vi "GenerateCalibrationSequence.vi"(8 "Pressure Group":u8[](array[numeric])=[3, 3, 3, 3, 4, 4, 4, 4], 11 "Mix Cluster":T1={"Ratio"=[0.6, 0.6, 0.6, 0.6, 0.6, 0.6, 0.6, 0.6], "Mix 2"=[8, 8], "Mix 1"=[0, 0]} {"Mix 1" items=["A1"=0, "A2"=1, "A3"=2, "A4"=3, "A5"=12]; "Mix 2" items=["B5"=8, "B6"=9, "B7"=10, "B8"=11, "A5"=12]}) -> (3 "Calibration Refs":T2)   [LabVIEW 2016]
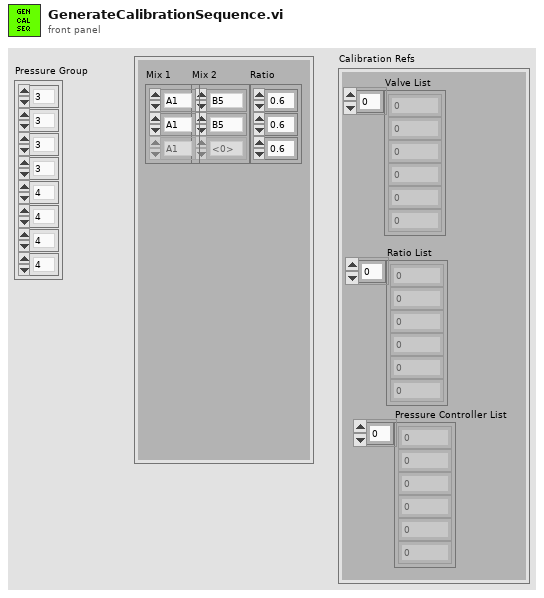
[diagram p1: front panel]
types:
  T1 = cluster{"Ratio":dbl[], "Mix 2":u16[], "Mix 1":u16[]}
  T2 = cluster{"Pressure Controller List":u8[], "Ratio List":dbl[], "Valve List":u16[]}
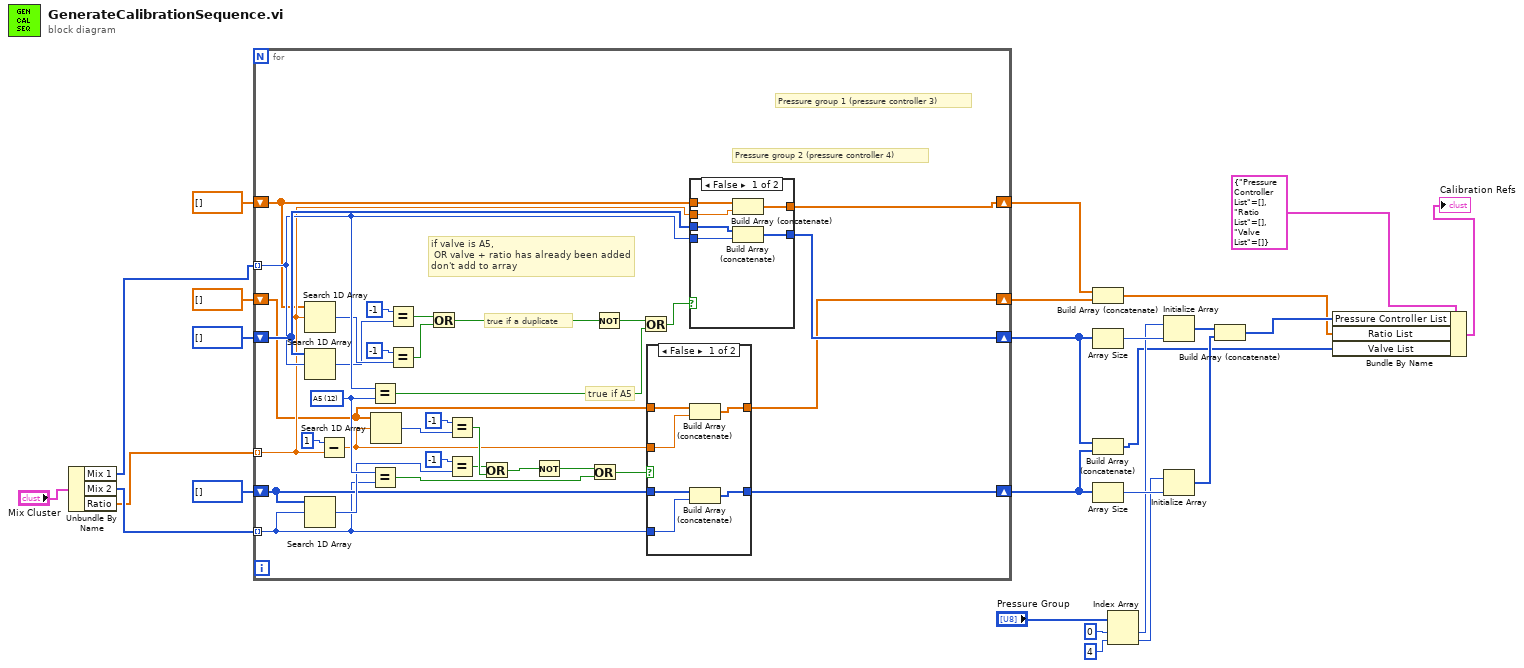
[diagram p0: block diagram]
diagram:
  n1 = Unbundle By Name("Mix Cluster") -> ("Mix 1"=w4:u16[], "Mix 2"=w3:u16[], "Ratio"=w2:dbl[])
  n2 = for {
    tunnel: w4 -> [w53] mode=indexing
    shift-right: [w60] -> w11
    shift-left: u16[] [] -> [w54]
    tunnel: w2 -> [w52] mode=indexing
    shift-right: [w56] -> w12
    shift-left: dbl[] [] -> [w51]
    tunnel: w3 -> [w33] mode=indexing
    shift-right: [w58] -> w13
    shift-left: dbl[] [] -> [w32]
    shift-right: [w57] -> w10
    shift-left: u16[] [] -> [w34]
    w55 = u16 12 items=["A1"=0, "A2"=1, "A3"=2, "A4"=3, "A5"=12] ("Ring")
    # "true if A5"
    # "true if a duplicate"
    # "if valve is A5,\n OR valve + ratio has already been added\ndon't add to array"
    # "Pressure group 2 (pressure controller 4)"
    # "Pressure group 1 (pressure controller 3)"
    n3 = Search 1D Array(1D array=w51, element=w52) -> (index of element=w50:i32)  [unwired: 1 in]
    n4 = Search 1D Array(1D array=w54, element=w53) -> (index of element=w49:i32)  [unwired: 1 in]
    n5 = Search 1D Array(1D array=w34, element=w33) -> (index of element=w40:i32)  [unwired: 1 in]
    n6 = Subtract(x=1, y=w52) -> (x-y=w31:dbl)
    n7 = Equal?(x=w53, y=w55) -> (x = y?=w43:bool)
    n8 = Equal?(x=w55, y=w33) -> (x = y?=w27:bool)
    n9 = Search 1D Array(1D array=w32, element=w31) -> (index of element=w41:i32)  [unwired: 1 in]
    n10 = Equal?(x=-1, y=w49) -> (x = y?=w45:bool)
    n11 = Equal?(x=-1, y=w50) -> (x = y?=w46:bool)
    n12 = Or(x=w45, y=w46) -> (x .or. y?=w44:bool)
    n13 = Equal?(x=-1, y=w41) -> (x = y?=w37:bool)
    n14 = Equal?(x=-1, y=w40) -> (x = y?=w36:bool)
    n15 = Or(x=w36, y=w37) -> (x .or. y?=w35:bool)
    n16 = Not(x=w35) -> (.not. x?=w28:bool)
    n17 = Or(x=w28, y=w27) -> (x .or. y?=w30:bool)
    n18 = Not(x=w44) -> (.not. x?=w29:bool)
    n19 = Or(x=w29, y=w43) -> (x .or. y?=w42:bool)
    n20 = case shown="False" w30 {
      tunnel: w33 -> [w66 _]
      tunnel: w34 -> [w65 w68]
      tunnel: [w64 w68] -> w57
      tunnel: w31 -> [w63 _]
      tunnel: w32 -> [w62 w67]
      tunnel: [w61 w67] -> w58
      frame False {
        n21 = Build Array (concatenate)(w62, w63) -> (w61:dbl[])
        n22 = Build Array (concatenate)(w65, w66) -> (w64:u16[])
      }
      frame True {
      }
    }
    n23 = case shown="False" w42 {
      tunnel: w53 -> [w74 _]
      tunnel: w54 -> [w73 w76]
      tunnel: [w72 w76] -> w60
      tunnel: w52 -> [w71 _]
      tunnel: w51 -> [w70 w75]
      tunnel: [w69 w75] -> w56
      frame False {
        n24 = Build Array (concatenate)(w70, w71) -> (w69:dbl[])
        n25 = Build Array (concatenate)(w73, w74) -> (w72:u16[])
      }
      frame True {
      }
    }
  }
  n26 = Build Array (concatenate)(w12, w13) -> (w7:dbl[])
  n27 = Array Size(array=w11) -> (size(s)=w21:i32)
  n28 = Build Array (concatenate)(w11, w10) -> (w6:u16[])
  n29 = Array Size(array=w10) -> (size(s)=w22:i32)
  n30 = Index Array(array="Pressure Group", index #1=0 ("index"), index #2=4 ("index")) -> (element #1=w19:u8, element #2=w17:u8)
  n31 = Initialize Array(w19, w21) -> (w16:u8[])
  n32 = Initialize Array(w17, w22) -> (w15:u8[])
  n33 = Build Array (concatenate)(w16, w15) -> (w8:u8[])
  n34 = Bundle By Name(cluster=T2 {"Pressure Controller List"=[], "Ratio List"=[], "Valve List"=[]} ("Calibration Refs"), "Pressure Controller List"=w8, "Ratio List"=w7, "Valve List"=w6) -> (→"Calibration Refs":T2)
